vi "GetLog.vi"(8 "Error in (no error)":errorcluster, 11 "Log in":refnum<class "Log.lvclass">) -> (0 "Error out":errorcluster, 2 "Array log out":T1[](array[typedef]) {"Priority" items=["EMERGENCY", "ALERT", "CRITICAL", "ERROR", "WARNING", "NOTICE", "INFO", "DEBUG"]}, 3 "Log out":refnum<class "Log.lvclass">)   [LabVIEW 2011, in "Log.lvclass"]
uses:
  Log.lvclass
  LogCluster.ctl
  PrioritiesRing.ctl
  Writer/LogWriterMock/LogWriterMock.lvclass
  Log.lvclass/Log.ctl
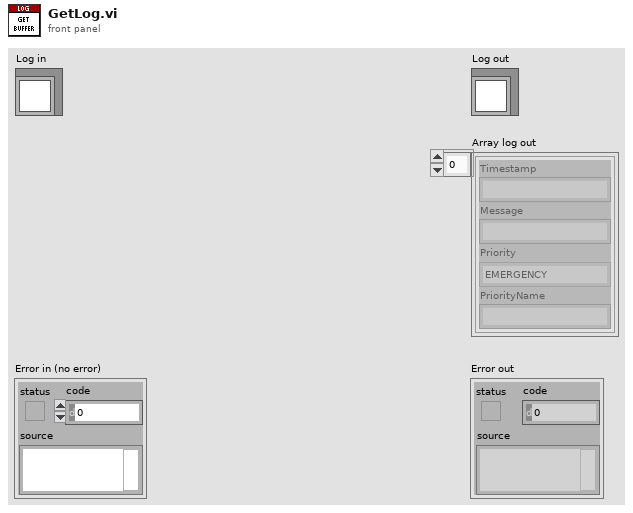
[diagram p1: front panel]
types:
  T1 = typedef "Log.lvclass/LogCluster.ctl" = cluster{"Timestamp":string, "Message":string, "Priority":T2, "PriorityName":string}
  T2 = typedef "Log.lvclass/PrioritiesRing.ctl" = u32
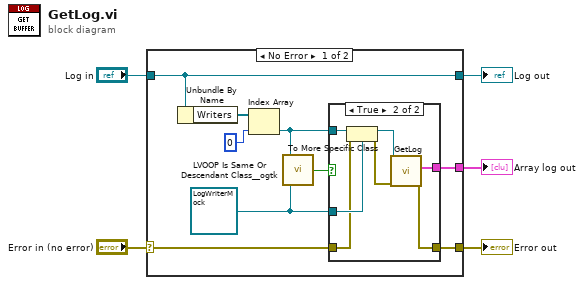
[diagram p0: block diagram]
diagram:
  n1 = case shown="No Error" "Error in (no error)" {
    selector: "Error in (no error)" -> [w6 w23]
    tunnel: [w12 w23] -> w4
    tunnel: [w14 w24] -> w2
    tunnel: "Log in" -> [w14 w24]
    tunnel: [w7 _] -> w1
    frame No Error {
      w8 = refnum<class "LogWriterMock.lvclass"> refnum ("LogWriterMock.lvclass")
      n2 = Unbundle By Name(w14) -> ("Writers"=w13:refnum<class "LogWriterInterface.lvclass">[])
      n3 = Index Array(array=w13, index=0) -> (element=w9:refnum<class "LogWriterInterface.lvclass">)
      n4 = call <userlib>:"LVOOP Is Same Or Descendant Class__ogtk.vi"("Possible Descendant Object"=w8, "Object"=w9) -> ("Is Same Class or Descendant?"=w10:bool)
      n5 = case shown="True" w10 {
        tunnel: [w15 w22] -> w12
        tunnel: w9 -> [_ w21]
        tunnel: w8 -> [_ w20]
        tunnel: [_ w18] -> w7
        tunnel: w6 -> [w15 w17]
        frame False {
        }
        frame True {
          n6 = To More Specific Class(target class=w20, reference=w21, error in=w17) -> (specific class reference=w19:refnum<class "LogWriterMock.lvclass">, error out=w16:errorcluster)
          n7 = call "GetLog.vi"("Error in (no error)"=w16, "LogWriterMock in"=w19) -> ("Error out"=w22:errorcluster, "Array log out"=w18:T1[])  [unwired: 7 in, 1 out]
        }
      }
    }
    frame Error {
    }
  }
  "Error out" <- w4
  "Log out" <- w2
  "Array log out" <- w1
